vi "Send ConfigureSpectrum.vi"(6 "Resolution BW":dbl=520.0 caption="Resolution BW (MHz)", 7 "Message Priority (Normal)":T1=enum."Normal", 8 "error in (no error)":errorcluster, 9 "center frequency":dbl=520.0 caption="Center Frequency (MHz)", 10 "span":dbl=1000.0 caption="Frequency span (MHz)", 11 "Message Enqueuer":refnum<class "Message Enqueuer.lvclass">) -> (0 "error out":errorcluster, 3 "Message Enqueuer out":refnum<class "Message Enqueuer.lvclass">)   [LabVIEW 2023, in "SpectrumAnalyzerInterface.lvlib" / "ConfigureSpectrum Msg.lvclass"]
doc: "This VI sends the message to an actor."
uses:
  ConfigureSpectrum Msg.lvclass
  <vilib>/ActorFramework/Message Enqueuer/Message Enqueuer.lvclass
  <vilib>/ActorFramework/Message Enqueuer/Message Priority.ctl
  ConfigureSpectrum Msg.lvclass/ConfigureSpectrum Msg.ctl
  <vilib>/ActorFramework/Message Enqueuer/Message Enqueuer.lvclass/Message Enqueuer.ctl
  <vilib>/ActorFramework/Message Priority Queue/Priority Enqueue.vi
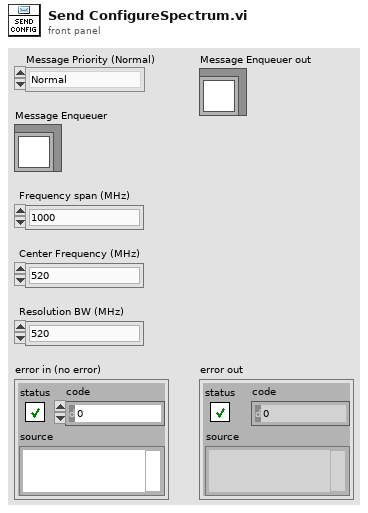
[diagram p1: front panel]
types:
  T1 = typedef "Actor Framework.lvlib/Message Enqueuer.lvclass/Message Priority.ctl" = enum16{"Low", "Normal", "High"}
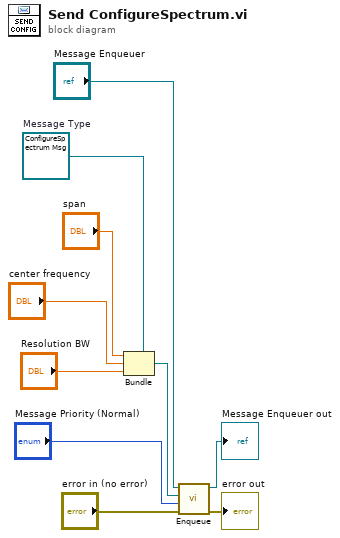
[diagram p0: block diagram]
diagram:
  w7 = refnum<class "ConfigureSpectrum Msg.lvclass"> refnum  # Message Type
  n1 = Bundle(cluster=w7, "span", "center frequency", "Resolution BW") -> (w6:refnum<class "ConfigureSpectrum Msg.lvclass">)
  n2 = call <vilib>:"Enqueue.vi"("error in (no error)"="error in (no error)", "Message Priority (Normal)"="Message Priority (Normal)", "Message"=w6, "Message Enqueuer in"="Message Enqueuer") -> ("error out"=→"error out":errorcluster, "Message Enqueuer out"=→"Message Enqueuer out":refnum<class "Message Enqueuer.lvclass">)  [unwired: 6 in]
